vi "test_2d_array.vi"() -> ()   [LabVIEW 2016]
panel:
  in  "Array":dbl[][](array[numeric])=[[1.0, 2.0], [4.0, 3.0], [5.0, 6.0]]
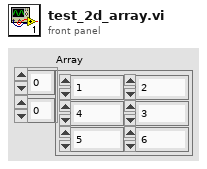
[diagram p1: front panel]
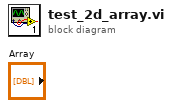
[diagram p0: block diagram]
diagram:
